vi "ConstructorString.vi"(6 "error in":errorcluster, 9 "CaseStructure in":refnum<class "CaseStructure.lvclass">) -> (0 "error out":errorcluster, 3 "CaseStructure out":refnum<class "CaseStructure.lvclass">, 4 "constructor":string)   [LabVIEW 2014, in "CaseStructure.lvclass"]
uses:
  CaseStructure.lvclass
  Python/Parsing/ListTypesTD.ctl
  Python/Parsing/Python Functions.lvlib
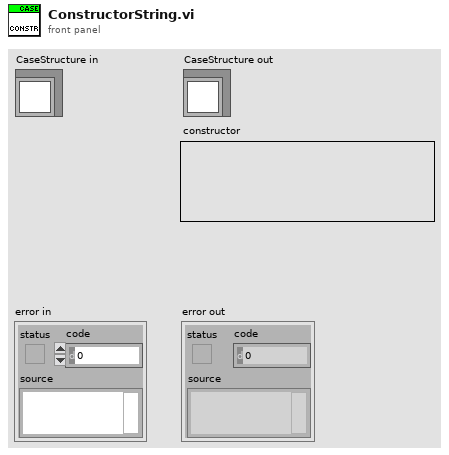
[diagram p1: front panel]
types:
  T1 = typedef "Python Functions.lvlib/ListTypesTD.ctl" = enum16{"list", "tuple", "parameter list", "output list"}
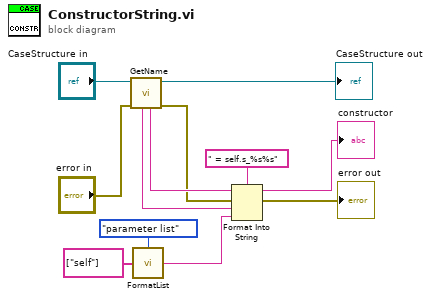
[diagram p0: block diagram]
diagram:
  n1 = call-dynamic "GetName.vi"("error in"="error in", "CaseStructure in"="CaseStructure in") -> ("error out"=w2:errorcluster, "CaseStructure out"=→"CaseStructure out":refnum<class "CaseStructure.lvclass">, "name"=w7:string, "UID"=w4:string)  [unwired: 4 in]
  n2 = call "FormatList.vi"("values"=string[] ["self"], "type"=ListTypesTD."parameter list") -> ("python object"=w5:string)
  n3 = Format Into String(format string=" = self.s_%s%s", initial string=w7, error in=w2, w4, w5) -> (resulting string=→"constructor":string, error out=→"error out":errorcluster)
